vi "practica_1.vi"() -> ()   [LabVIEW 2025]
panel:
  out "Result":string
  in  "Numeric 4":dbl
  in  "Numeric 3":dbl
  in  "Numeric 2":dbl
  in  "Numeric":dbl
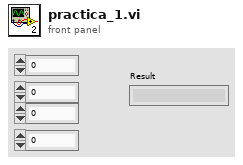
[diagram p1: front panel]
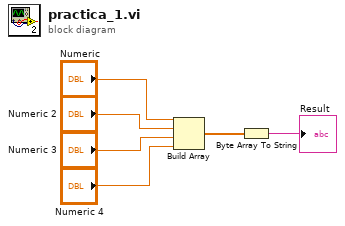
[diagram p0: block diagram]
diagram:
  n1 = Build Array("Numeric", "Numeric 2", "Numeric 3", "Numeric 4") -> (w2:dbl[])
  n2 = Byte Array To String(unsigned byte array=w2) -> (string=→"Result":string)
